vi "PM.TestLauncher.vi"() -> ()   [LabVIEW 2017, in "OPM.lvclass"]
doc: "JKI State Machine Objects (SMO) 1.0.0.5\nJKI - JKI\nCopyright (c) 2016, JKI"
uses:
  OPM.lvclass
  <vilib>/JKI/JKI SMO/SMO/Typedefs/SMOState --Enum.ctl
  OPM.ThorlabsPM400/OPM.ThorlabsPM400.lvclass
  OPM.Simulated/OPM.Simulated.lvclass
  D:/upwork/Laser Measurement Tool/Laser/project/Subsystems/OPM/OPM.lvclass
  D:/Program Files (x86)/National Instruments/LabVIEW 2017/vi.lib/JKI/JKI SMO/SMO/SMO.lvclass
  D:/upwork/Laser Measurement Tool/Laser/project/Subsystems/MeasuringDevice/MeasuringDevice.lvclass
  <vilib>/JKI/JKI SMO/SMO/SMO.lvclass
  MeasuringDevice/MeasuringDevice.lvclass
panel:
  out "Power, W":dbl
  in  "Measure Button":bool
  out "SMO State":T1
  out "error out":errorcluster
  in  "Stop":bool
  # "OPM Test Launcher"
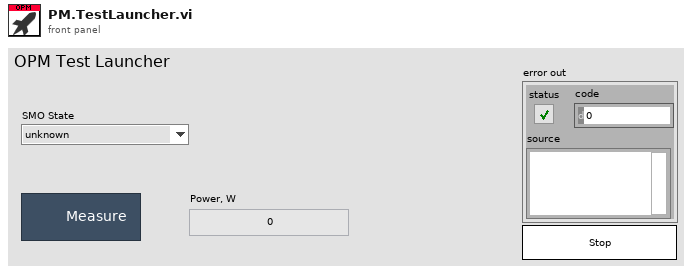
[diagram p1: front panel]
types:
  T1 = typedef "SMO.lvclass/SMOState --Enum.ctl" = enum16{"unknown", "Created", "Started", "Stopped"}
  T2 = typedef "SMO.lvclass/Public Events.ctl" = cluster{"Error":refnum<user-event>, "State":refnum<user-event>, "Reserve State":refnum<user-event>}
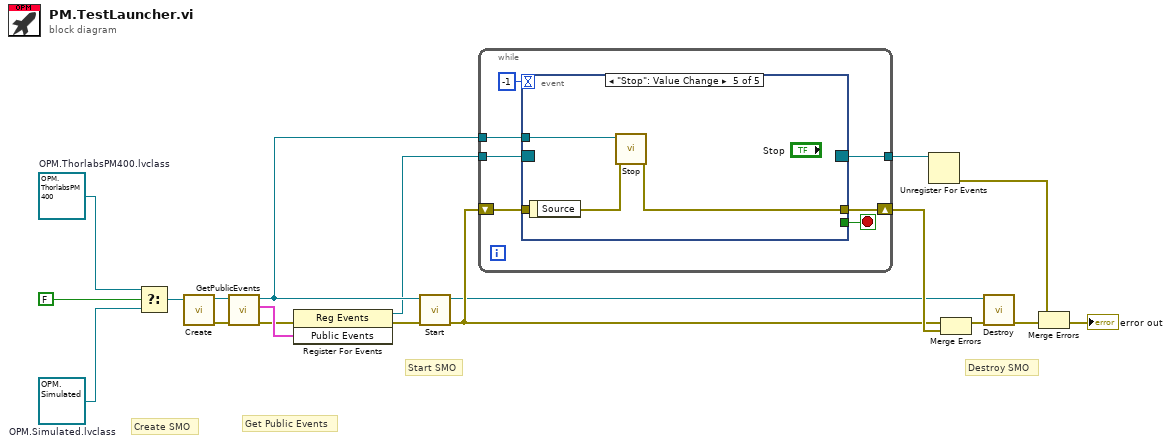
[diagram p0: block diagram]
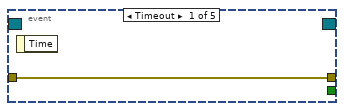
[diagram p2: hidden frame]
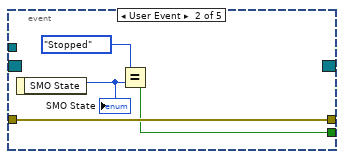
[diagram p3: hidden frame]
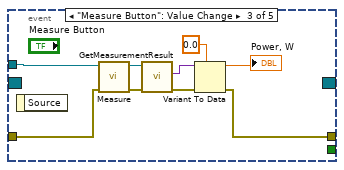
[diagram p4: hidden frame]
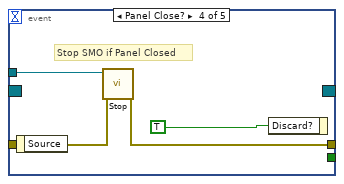
[diagram p5: hidden frame]
diagram:
  w3 = refnum<class "OPM.Simulated.lvclass"> refnum  # OPM.Simulated.lvclass
  w4 = refnum<class "OPM.ThorlabsPM400.lvclass"> refnum  # OPM.ThorlabsPM400.lvclass
  # "Get Public Events"
  # "Start SMO"
  # "Destroy SMO"
  # "Create SMO"
  n1 = Select(t=w4, s=FALSE, f=w3) -> (s? t:f=w2:refnum<class "OPM.lvclass">)
  n2 = call <vilib>:"Create.vi"("SMO"=w2) -> ("error out"=w5:errorcluster, "SMO out"=w6:refnum<class "OPM.lvclass">)  [unwired: 8 in, 1 out]
  n3 = call <vilib>:"GetPublicEvents.vi"("error in (no error)"=w5, "SMO"=w6) -> ("error out"=w8:errorcluster, "Public Events"=w9:T2, "SMO out"=w11:refnum<class "OPM.lvclass">)  [unwired: 7 in]
  n4 = register-events(error in=w8, w9) -> (reference out=w7:refnum<event-registration>, error out=w10:errorcluster)  [unwired: 1 in]
  n5 = call <vilib>:"Start.vi"("error in (no error)"=w10, "SMO"=w11) -> ("error out"=w14:errorcluster, "SMO out"=w12:refnum<class "OPM.lvclass">)  [unwired: 8 in]
  n6 = while {
    shift-right: [w25] -> w18
    shift-left: w14 -> [w24]
    tunnel: w7 -> [w23]
    tunnel: [w22] -> w19
    tunnel: w11 -> [w21]
    stop <- w26 stop-if-true
    n7 = event shown="[4] \"Stop\": Value Change" {
      selector: w23 -> [_ _ _ _ _]
      dyn-events: [_ _ _ _ _] -> w22
      timeout: -1 -> [_ _ _ _ _]
      tunnel: [_ w28 _ _ _] -> w26
      tunnel: w21 -> [_ _ w40 w44 w47]
      tunnel: [w27 w31 w33 w43 w46] -> w25
      tunnel: w24 -> [w27 w31 w39 w42 w45]
      event Timeout {
        n8 = event-data() -> ()  [unwired: 1 in, 1 out]
      }
      event User Event {
        n9 = event-data() -> ("SMO State"=w30:T1)  [unwired: 1 in]
        "SMO State" <- w30
        n10 = Equal?(x=SMOState_--Enum."Stopped", y=w30) -> (x = y?=w28:bool)
      }
      event "Measure Button": Value Change {
        n11 = event-data() -> ()  [unwired: 1 in, 1 out]
        n12 = call "Measure.vi"("error in (no error)"=w39, "MeasuringDevice"=w40) -> ("error out"=w37:errorcluster, "MeasuringDevice out"=w38:refnum<class "OPM.lvclass">)  [unwired: 7 in, 1 out]
        n13 = call "GetMeasurementResult.vi"("error in (no error)"=w37, "MeasuringDevice in"=w38) -> ("error out"=w35:errorcluster, "Result"=w36:variant)  [unwired: 7 in, 1 out]
        n14 = Variant To Data(error in=w35, type=0.0, Variant=w36) -> (data=→"Power, W":dbl, error out=w33:errorcluster)
      }
      event Panel Close? {
        # "Stop SMO if Panel Closed"
        n15 = event-data() -> ()  [unwired: 1 in, 1 out]
        n16 = call <vilib>:"Stop.vi"("error in (no error)"=w42, "SMO"=w44) -> ("error out"=w43:errorcluster)  [unwired: 8 in, 1 out]
        n17 = event-data("Discard?"=TRUE ("OK")) -> ()  [unwired: 1 in, 1 out]
      }
      event "Stop": Value Change {
        n18 = event-data() -> ()  [unwired: 1 in, 1 out]
        n19 = call <vilib>:"Stop.vi"("error in (no error)"=w45, "SMO"=w47) -> ("error out"=w46:errorcluster)  [unwired: 8 in, 1 out]
      }
    }
  }
  n20 = Unregister For Events(event registration refnum=w19) -> (error out=w17:errorcluster)  [unwired: 1 in]
  n21 = Merge Errors(w14, w18) -> (w13:errorcluster)
  n22 = call <vilib>:"Destroy.vi"("error in (no error)"=w13, "SMO"=w12) -> ("error out"=w15:errorcluster)  [unwired: 9 in]
  n23 = Merge Errors(w17, w15) -> (→"error out":errorcluster)
